vi "Elevator State Select.vi"() -> (0 "Elevator_State":string)   [LabVIEW 2018]
uses:
  RefNumsDriverStation.vi
  Robot States.vi
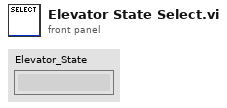
[diagram p1: front panel]
types:
  T1 = cluster{"Elevator_Stow":bool, "Cargo_Rocket_1":bool, "Hatch_Rocket_1":bool, "Cargo_Ground":bool, "Hatch_Feeder":bool, "Cargo_Ship":bool, "Hatch_Ship":bool}
  T2 = cluster{"Trigger":bool, "Trigger":bool, "Trigger":bool, "Trigger":bool, "Trigger":bool, "Trigger":bool, "Trigger":bool}
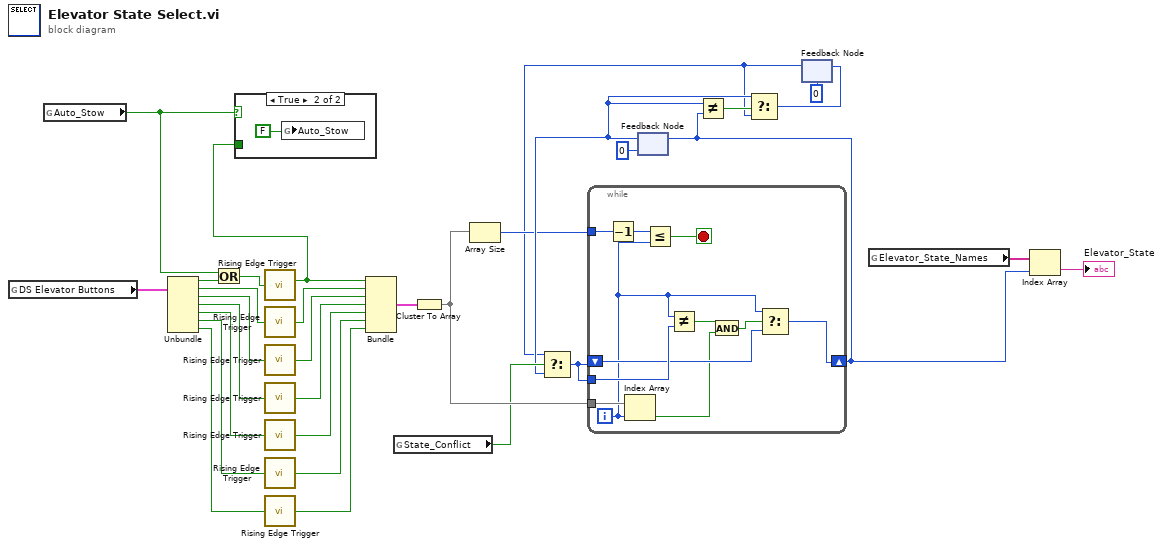
[diagram p0: block diagram]
diagram:
  n1 = global read "RefNumsDriverStation.vi" "DS Elevator Buttons"() -> (w31:T1)
  n2 = global read "Robot States.vi" "Auto_Stow"() -> (w15:bool)
  n3 = Unbundle(w31) -> ("Elevator_Stow"=w17:bool, "Cargo_Rocket_1"=w30:bool, "Hatch_Rocket_1"=w29:bool, "Cargo_Ground"=w28:bool, "Hatch_Feeder"=w27:bool, "Cargo_Ship"=w26:bool, "Hatch_Ship"=w25:bool)
  n4 = Or(x=w15, y=w17) -> (x .or. y?=w16:bool)
  n5 = call "Rising Edge Trigger.vi"("Raw Signal"=w16) -> ("Trigger"=w14:bool)
  n6 = case shown="True" w15 {
    tunnel: w14 -> [_ _]
    frame False {
    }
    frame True {
      n7 = global write "Robot States.vi" "Auto_Stow"(FALSE ("Auto_Stow")) -> ()
    }
  }
  n8 = call "Rising Edge Trigger.vi"("Raw Signal"=w30) -> ("Trigger"=w24:bool)
  n9 = call "Rising Edge Trigger.vi"("Raw Signal"=w29) -> ("Trigger"=w23:bool)
  n10 = call "Rising Edge Trigger.vi"("Raw Signal"=w28) -> ("Trigger"=w22:bool)
  n11 = call "Rising Edge Trigger.vi"("Raw Signal"=w27) -> ("Trigger"=w21:bool)
  n12 = call "Rising Edge Trigger.vi"("Raw Signal"=w26) -> ("Trigger"=w20:bool)
  n13 = call "Rising Edge Trigger.vi"("Raw Signal"=w25) -> ("Trigger"=w19:bool)
  n14 = Bundle("Trigger"=w14, "Trigger"=w24, "Trigger"=w23, "Trigger"=w22, "Trigger"=w21, "Trigger"=w20, "Trigger"=w19) -> (w18:T2)  [unwired: 1 in]
  n15 = global read "Robot States.vi" "State_Conflict"() -> (w12:bool)
  n16 = Cluster To Array(cluster=w18) -> (array=w13:bool[])
  n17 = Array Size(array=w13) -> (size(s)=w8:i32)
  n18 = feedback #1(0) -> (w10:i32)
  n19 = feedback #2(0) -> (w2:i32)
  n20 = Select(t=w2, s=w12, f=w10) -> (s? t:f=w9:i32)
  n21 = while {
    tunnel: w13 -> [w43]
    shift-right: [w35] -> w7
    shift-left: w9 -> [w36]
    tunnel: w9 -> [w40]
    tunnel: w8 -> [w39]
    i -> [w34]
    stop <- w37 stop-if-true
    n22 = Decrement(x=w39) -> (x-1=w38:i32)
    n23 = Index Array(array=w43, index=w34) -> (element=w33:bool)
    n24 = Less Or Equal?(x=w38, y=w34) -> (x <= y?=w37:bool)
    n25 = Not Equal?(x=w34, y=w40) -> (x != y?=w42:bool)
    n26 = And(x=w42, y=w33) -> (x .and. y?=w41:bool)
    n27 = Select(t=w34, s=w41, f=w36) -> (s? t:f=w35:i32)
  }
  n28 = feedback-in #1(w7) -> ()
  n29 = Not Equal?(x=w10, y=w7) -> (x != y?=w11:bool)
  n30 = Select(t=w10, s=w11, f=w2) -> (s? t:f=w6:i32)
  n31 = feedback-in #2(w6) -> ()
  n32 = global read "Robot States.vi" "Elevator_State_Names"() -> (w4:string[])
  n33 = Index Array(array=w4, index=w7) -> (element=→"Elevator_State":string)
